vi "IRCalibrationTest.vi"() -> ()   [LabVIEW 2019]
uses:
  <vilib>/Platform/TimedLoop/XDataNode/timing_clust.ctl
  <vilib>/Platform/TimedLoop/XDataNode/nitl_modes.ctl
  <vilib>/Platform/TimedLoop/XDataNode/wakeup.ctl
  WSCbot_V3_Toolkit.lvlibp/WSCBOTV3_Toolkit/Sensor/LowLevel/IR_Chanel.ctl
  WSCbot_V3_Toolkit.lvlibp/WSCBOTV3_Toolkit/Sensor/LowLevel/InfraredRanging(Array).vi
  <vilib>/addons/control/pid/pid.llb/PID (DBL).vi
  WSCbot_V3_Toolkit.lvlibp/WSCBOTV3_Toolkit/System/LowLevel/Buzzer.vi
  <vilib>/platform/TimedLoop/XDataNode/XDataNode.xnode
  <vilib>/Platform/TimedLoop/XDataNode/XDNodeRunTimeDep.lvlib
  WSCbot_V3_Toolkit.lvlibp
  <vilib>/ptbypt/NI_PtbyPt.lvlib
  <vilib>/addons/control/pid/NI_PID_pid.lvlib
panel:
  in  "USdis":dbl=300.0 format="%#_13g"
  in  "P 2":dbl
  out "error":cluster{dbl, dbl, dbl}(graph)
  in  "P":dbl
  out "Waveform Chart 2":T1(graph)
  out "Waveform Chart":T2(graph)
  in  "Stop Button":bool
  out "Distance_L(mm)":dbl
  out "Distance_R(mm)":dbl
  out "Valtage":dbl[](array[numeric])
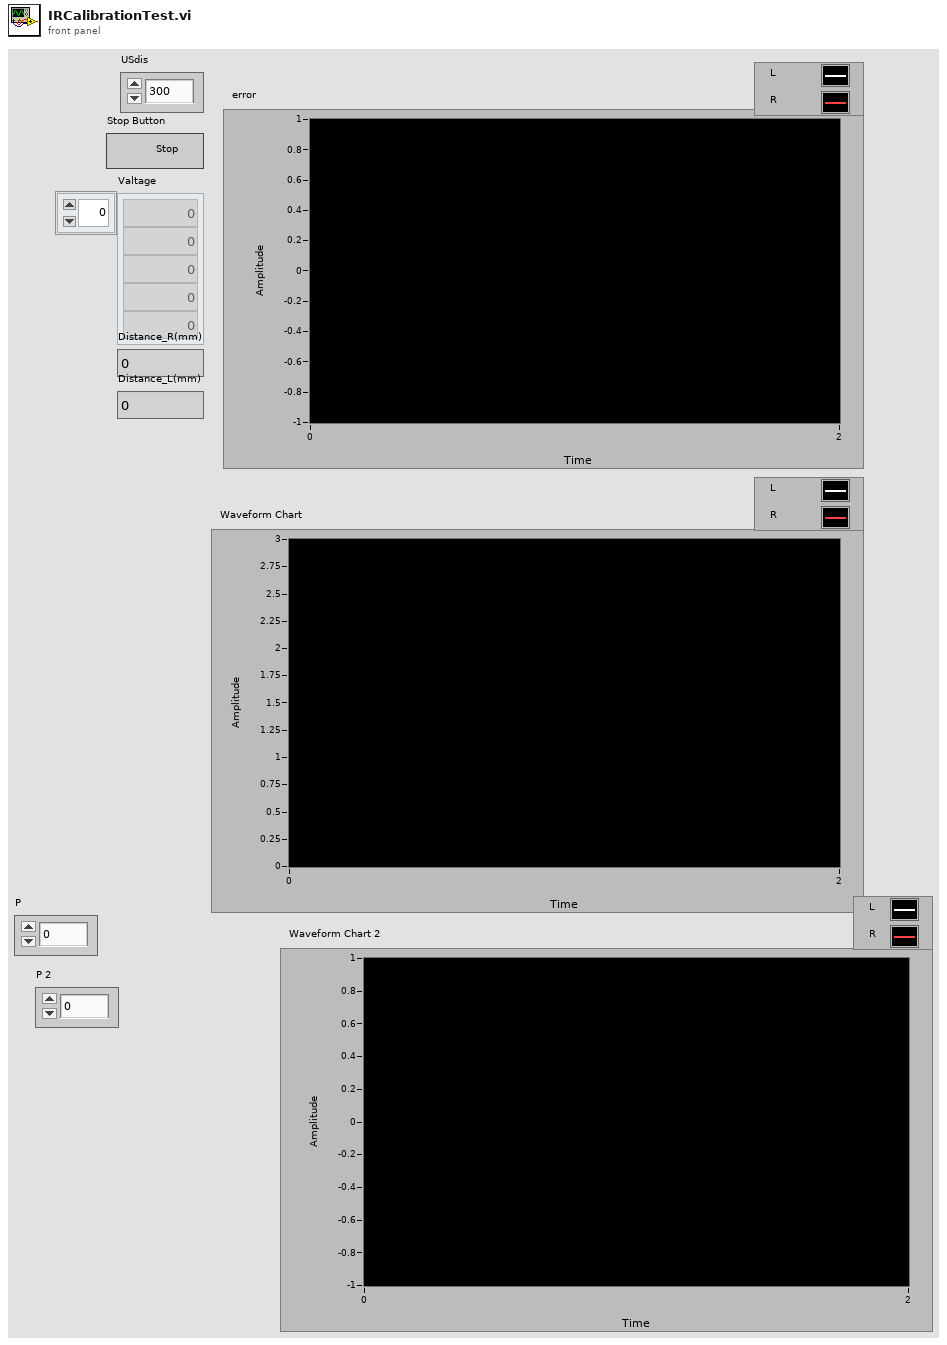
[diagram p1: front panel]
types:
  T1 = cluster{"Distance_L(mm)":dbl, "Distance_R(mm)":dbl}
  T2 = cluster{"Valtage[0]":dbl, "Valtage[1]":dbl, "Valtage[2]":dbl, "Valtage[3]":dbl, "Valtage[4]":dbl, "Valtage[5]":dbl, "Valtage[6]":dbl, "Valtage[7]":dbl, "Valtage[8]":dbl}
  T3 = typedef "XDNodeRunTimeDep.lvlib/timing_clust.ctl" = cluster{"Expected End [f-1]":u64, "Actual End [f-1]":u64, "Finished Late? [f-1]":bool, "Expected End [i-1]":u64, "Actual End [i-1]":u64, "Finished Late? [i-1]":bool, "Expected Start [i]":u64, "Actual Start [i]":u64, "Expected Start [f]":u64, "Actual Start [f]":u64, "Source Name":string, "Structure Name":string, "Period":i64, "Deadline":i64, "Offset":i64, "Start":i64, "Priority":i32, "Timeout":i32, "Mode":T4, "Wakeup Reason":T5, "Error":errorcluster, "Source Type":string, "Secondary Source Type":string, "Global End Time":u64, "Global Start Time":u64, "Frame Duration":u64, "Iteration Duration":u64, "Assigned CPU":i32, "I/O Scan Engine Mode":u32}
  T4 = typedef "XDNodeRunTimeDep.lvlib/nitl_modes.ctl" = enum32{"No Change", "Process missed periods, maintain original phase", "Discard missed periods, maintain original phase", "Process missed periods, ignore original phase", "Discard missed periods, ignore original phase"}
  T5 = typedef "XDNodeRunTimeDep.lvlib/wakeup.ctl" = enum32{"Normal", "Aborted", "Asynchronous wakeup", "Timing source error", "Timed loop error", "Timeout"}
  T6 = cluster{"proportional gain (Kc)":dbl, "integral time (Ti, min)":dbl, "derivative time (Td, min)":dbl}
  T7 = typedef "WSCbot_V3_toolkit.lvlibp/IR_Chanel.ctl" = enum16{"IR_LF", "IR_LB", "IR_BL", "IR_BR", "IR_RB", "IR_RF", "IR_FR", "IR_FL"}
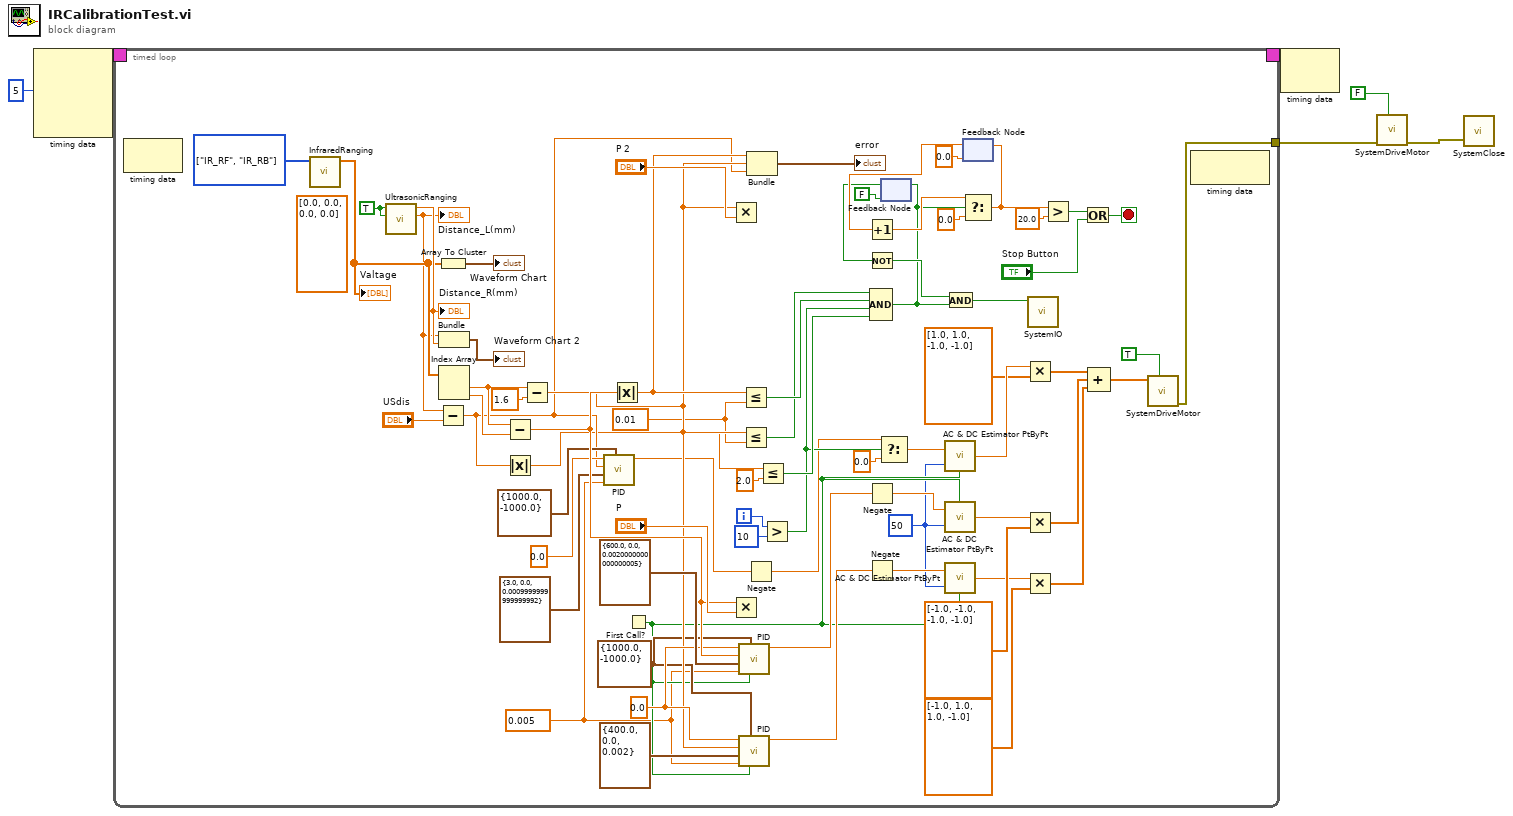
[diagram p0: block diagram]
diagram:
  n1 = node-c288(i64 5 ("Period")) -> (w6:T3)  [unwired: 3 in]
  n2 = timed-loop {
    timing: w6 -> [_]
    timing-out: [_] -> w5
    tunnel: [w65] -> w1
    i -> [w63]
    stop <- w61 stop-if-true
    w11 = 50 ("sample length")
    w26 = 0.005 ("dt (s)")
    w42 = cluster{"output high":dbl, "output low":dbl} {"output high"=1000.0, "output low"=-1000.0} ("output range")
    w45 = 0.0 ("setpoint")
    w22 = 0.01 ("y")
    w74 = T7[] [enum."IR_RF", enum."IR_RB"] items=["IR_LF", "IR_LB", "IR_BL", "IR_BR", "IR_RB", "IR_RF", "IR_FR", "IR_FL"] ("IR_Chanel")
    w77 = TRUE ("Enable_R")
    (unwired) dbl[] [0.0, 0.0, 0.0, 0.0] ("4xMotor(deg/s)")
    n3 = node-c288() -> ()  [unwired: 1 in, 1 out]
    n4 = call-poly "InfraredRanging.vi"("IR_Chanel"=w74) -> ("Valtage"=w72:dbl[])  [unwired: 9 in, 1 out]
    "Valtage" <- w72
    n5 = call "UltrasonicRanging.vi"("Enable_L"=w77, "Enable_R"=w77) -> ("Distance_L(mm)"=w29:dbl, "Distance_R(mm)"=w76:dbl)  [unwired: 7 in, 1 out]
    "Distance_R(mm)" <- w76
    "Distance_L(mm)" <- w29
    n6 = Array To Cluster(array=w72) -> (cluster=→"Waveform Chart":T2)
    n7 = Subtract(x=w29, y="USdis") -> (x-y=w18:dbl)
    n8 = Bundle("Distance_L(mm)"=w29, "Distance_R(mm)"=w76) -> (→"Waveform Chart 2":T1)  [unwired: 1 in]
    n9 = Index Array(array=w72) -> (element #1=w60:dbl, element #2=w71:dbl)  [unwired: 2 in]
    n10 = Subtract(x=w60, y=w71) -> (x-y=w49:dbl)
    n11 = Absolute Value(x=w18) -> (abs(x)=w17:dbl)
    n12 = Subtract(x=w60, y=1.6) -> (x-y=w44:dbl)
    n13 = call-poly <vilib>:"PID.vi"("output range"=cluster{"output high":dbl, "output low":dbl} {"output high"=1000.0, "output low"=-1000.0}, "dt (s)"=w26, "PID gains"=T6 {"proportional gain (Kc)"=3.0, "integral time (Ti, min)"=0.0, "derivative time (Td, min)"=0.0009999999999999992} ("PID gains 3"), "process variable"=w18, "setpoint"=0.0) -> ("output"=w23:dbl)  [unwired: 5 in, 1 out]
    n14 = Absolute Value(x=w49) -> (abs(x)=w51:dbl)
    n15 = First Call?() -> (First Call?: T/F=w30:bool)
    n16 = Multiply(x=w44, y="P 2") -> ()  [unwired: 1 out]
    n17 = Multiply(x=w49, y="P") -> ()  [unwired: 1 out]
    n18 = call-poly <vilib>:"PID.vi"("reinitialize? (F)"=w30, "output range"=w42, "dt (s)"=w26, "PID gains"=T6 {"proportional gain (Kc)"=600.0, "integral time (Ti, min)"=0.0, "derivative time (Td, min)"=0.0020000000000000005}, "process variable"=w49, "setpoint"=w45) -> ("output"=w47:dbl)  [unwired: 4 in, 1 out]
    n19 = call-poly <vilib>:"PID.vi"("reinitialize? (F)"=w30, "output range"=w42, "dt (s)"=w26, "PID gains"=T6 {"proportional gain (Kc)"=400.0, "integral time (Ti, min)"=0.0, "derivative time (Td, min)"=0.002} ("PID gains 2"), "process variable"=w44, "setpoint"=w45) -> ("output"=w41:dbl)  [unwired: 4 in, 1 out]
    n20 = Less Or Equal?(x=w51, y=w22) -> (x <= y?=w64:bool)
    n21 = Less Or Equal?(x=w44, y=w22) -> (x <= y?=w53:bool)
    n22 = Negate(x=w23) -> (-x=w9:dbl)
    n23 = Bundle(w51, w44, w18) -> (→"error":cluster{dbl, dbl, dbl})  [unwired: 1 in]
    n24 = Less Or Equal?(x=w17, y=2.0) -> (x <= y?=w20:bool)
    n25 = Greater?(x=w63, y=10) -> (0:w10:bool)
    n26 = Negate(x=w47) -> (-x=w46:dbl)
    n27 = Negate(x=w41) -> (-x=w40:dbl)
    n28 = Compound Arithmetic op=AND(w53, w64, w10, w20) -> (w12:bool)
    n29 = Select(t=w9, s=w10, f=0.0) -> (s? t:f=w7:dbl)
    n30 = feedback-in #1(w12) -> ()
    n31 = feedback #1(FALSE) -> (w15:bool)
    n32 = Not(x=w15) -> (.not. x?=w14:bool)
    n33 = call <vilib>:"AC & DC Estimator PtByPt.vi"("signal"=w7, "sample length"=w11, "initialize"=w30) -> ("DC estimate (V)"=w32:dbl)  [unwired: 2 out]
    n34 = call <vilib>:"AC & DC Estimator PtByPt.vi"("signal"=w46, "sample length"=w11, "initialize"=w30) -> ("DC estimate (V)"=w54:dbl)  [unwired: 2 out]
    n35 = call <vilib>:"AC & DC Estimator PtByPt.vi"("signal"=w40, "sample length"=w11, "initialize"=w30) -> ("DC estimate (V)"=w55:dbl)  [unwired: 2 out]
    n36 = And(x=w14, y=w12) -> (x .and. y?=w16:bool)
    n37 = feedback #2(0.0 ("f")) -> (w39:dbl)
    n38 = Increment(x=w39) -> (x+1=w38:dbl)
    n39 = Select(t=w38, s=w12, f=0.0) -> (s? t:f=w36:dbl)
    n40 = feedback-in #2(w36) -> ()
    n41 = Multiply(x=w32, y=dbl[] [1.0, 1.0, -1.0, -1.0] ("4xMotor(deg/s)")) -> (x*y=w19:dbl[])
    n42 = Multiply(x=w54, y=dbl[] [-1.0, -1.0, -1.0, -1.0] ("4xMotor(deg/s)")) -> (x*y=w68:dbl[])
    n43 = Multiply(x=w55, y=dbl[] [-1.0, 1.0, 1.0, -1.0] ("4xMotor(deg/s)")) -> (x*y=w56:dbl[])
    n44 = call-poly "SystemIO.vi"("Set"=w16) -> ()  [unwired: 10 in, 1 out]
    n45 = Greater?(x=w36, y=20.0) -> (0:w34:bool)
    n46 = Or(x=w34, y="Stop Button") -> (x .or. y?=w61:bool)
    n47 = Compound Arithmetic op=ADD(w19, w68, w56) -> (w67:dbl[])
    n48 = call "SystemDriveMotor.vi"("Enable?"=TRUE, "4xMotor(deg/s)"=w67) -> ("error out"=w65:errorcluster)  [unwired: 8 in, 1 out]
    n49 = node-c288() -> ()  [unwired: 1 in, 1 out]
  }
  n50 = node-c288(w5) -> ()  [unwired: 1 out]
  n51 = call "SystemDriveMotor.vi"("Enable?"=FALSE, "error in"=w1) -> ("error out"=w2:errorcluster)  [unwired: 8 in, 1 out]
  n52 = call "SystemClose.vi"("error in"=w2) -> ()  [unwired: 2 in, 1 out]
